vi "Run.vi"() -> ()   [LabVIEW 2019, in "UnitTestFramework.lvclass"]
uses:
  UnitTestFramework.lvclass
panel:
  out "Test Result":string
  out "error out":errorcluster
  in  "UnitTestFramework.lvclass":refnum<class "UnitTestFramework.lvclass">
  in  "Test Suit Path":path
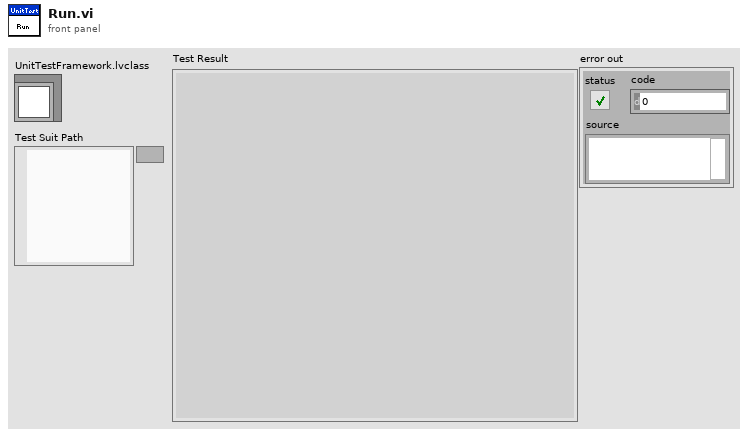
[diagram p1: front panel]
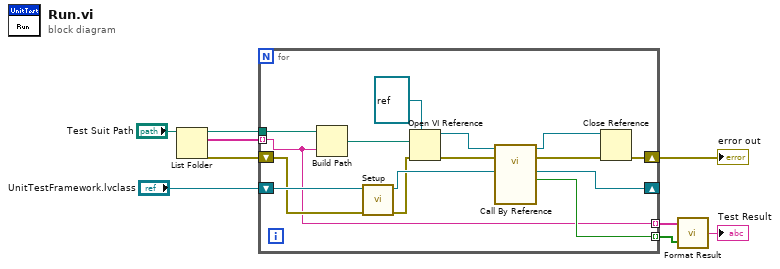
[diagram p0: block diagram]
diagram:
  n1 = List Folder(path="Test Suit Path") -> (path out=w8:path, filenames=w7:string[], error out=w6:errorcluster)  [unwired: 3 in, 1 out]
  n2 = for {
    tunnel: w8 -> [w24]
    tunnel: w7 -> [w10] mode=indexing
    shift-right: [w17] -> w4
    shift-left: w6 -> [w14]
    shift-right: [w12] -> _
    shift-left: "UnitTestFramework.lvclass" -> [w16]
    tunnel: [w11] -> w2 mode=indexing
    tunnel: [w10] -> w3 mode=indexing
    n3 = Build Path(base path=w24, name or relative path=w10) -> (appended path=w23:path)
    n4 = call-dynamic "Setup.vi"("error in (no error)"=w14, "UnitTestFramework in"=w16) -> ("error out"=w13:errorcluster, "UnitTestFramework out"=w15:refnum<class "UnitTestFramework.lvclass">)  [unwired: 8 in]
    n5 = Open VI Reference(type specifier VI Refnum (for type only)=refnum<vi> refnum, vi path=w23, error in (no error)=w13) -> (vi reference=w20:refnum<vi>, error out=w21:errorcluster)  [unwired: 3 in]
    n6 = call-by-ref "?"(reference=w20, error in=w21, "UnitTestFramework.lvclass in"=w15) -> (reference out=w18:refnum<vi>, error out=w19:errorcluster, "Equal?"=w11:bool, "UnitTestFramework.lvclass out"=w12:refnum<class "UnitTestFramework.lvclass">)  [unwired: 8 in, 1 out]
    n7 = Close Reference(reference=w18, error in (no error)=w19) -> (error out=w17:errorcluster)
  }
  "error out" <- w4
  n8 = call "Format Result.vi"("Pass?"=w2, "VI names"=w3) -> ("Result"=→"Test Result":string)
